vi "relay_block5.vi"(8 "error in":errorcluster, 11 "Modbus master in":refnum<class "Modbus Master.lvclass">) -> (0 "error out":errorcluster, 3 "Modbus master out":refnum<class "Modbus Master.lvclass">)   [LabVIEW 2020]
uses:
  <vilib>/NI/Modbus Library/API/Master/Modbus Master.lvclass
  C:/Program Files/National Instruments/LabVIEW 2020/vi.lib/NI/Modbus Library/API/Modbus API.lvclass
  <vilib>/NI/Modbus Library/API/Modbus API.lvclass/Modbus API.ctl
  <vilib>/NI/Modbus Library/Transmission Data Unit/Transmission Data Unit.lvclass/Transmission Data Unit.ctl
  <vilib>/NI/Modbus Library/Transmission Data Unit/Write Unit ID.vi
  <vilib>/NI/Modbus Library/API/Read Transmission Data Unit.vi
  <vilib>/NI/Modbus Library/API/Write Transmission Data Unit.vi
  status/emergency stop.vi
panel:
  out "current time":timestamp
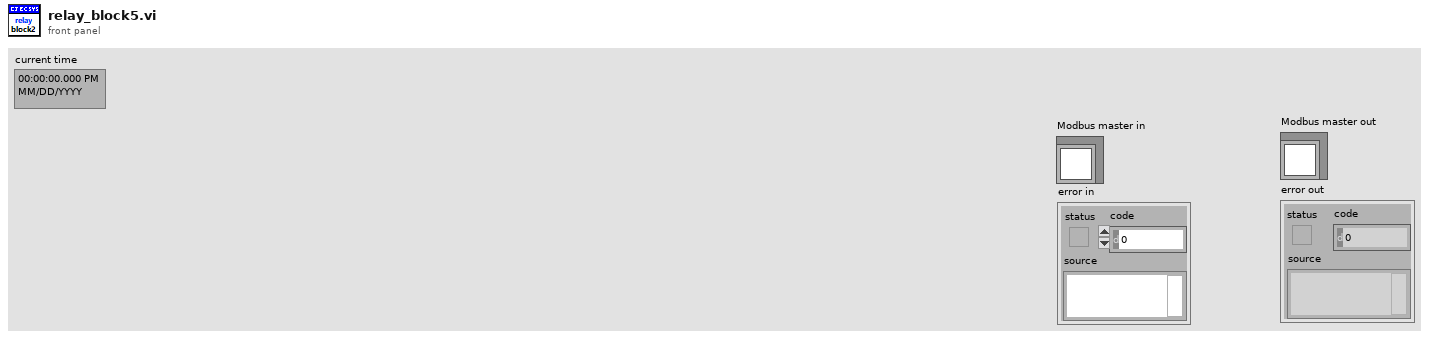
[diagram p1: front panel]
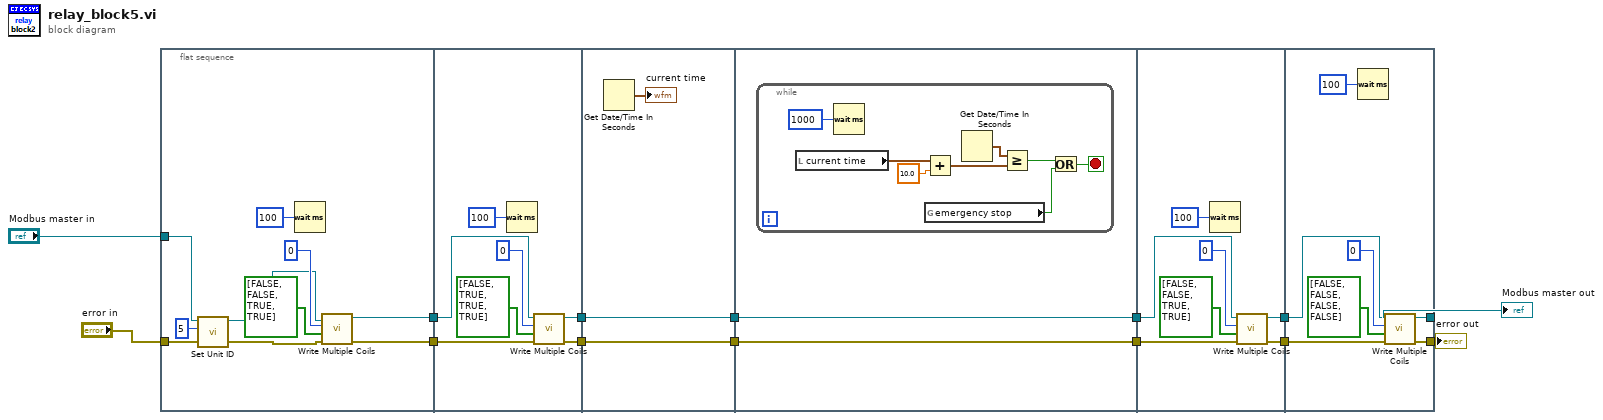
[diagram p0: block diagram]
diagram:
  n1 = flat-sequence {
    tunnel: "error in" -> [w19]
    tunnel: "Modbus master in" -> [w18]
    tunnel: [w21] -> w12
    tunnel: [w20] -> w11
    tunnel: w12 -> [w28]
    tunnel: w11 -> [w27]
    tunnel: [w26] -> w10
    tunnel: [w25] -> w5
    tunnel: w10 -> [w33]
    tunnel: [w33] -> w9
    tunnel: [w32] -> w6
    tunnel: w5 -> [w32]
    tunnel: w9 -> [w36]
    tunnel: [w36] -> w8
    tunnel: [w35] -> w7
    tunnel: w6 -> [w35]
    tunnel: w8 -> [w48]
    tunnel: w7 -> [w47]
    tunnel: [w46] -> w4
    tunnel: [w45] -> w3
    tunnel: w4 -> [w55]
    tunnel: w3 -> [w54]
    tunnel: [w53] -> w2
    tunnel: [w52] -> w1
    frame #0 {
      n2 = call <vilib>:"Set Unit ID.vi"("error in"=w19, "unit ID"=u8 5, "Modbus master in"=w18) -> ("error out"=w16:errorcluster, "Modbus master out"=w17:refnum<class "Modbus Master.lvclass">)  [unwired: 7 in]
      n3 = Wait (ms)(milliseconds to wait=u32 100) -> ()  [unwired: 1 out]
      n4 = call-dynamic "Write Multiple Coils.vi"("error in"=w16, "coils to write"=bool[] [FALSE, FALSE, TRUE, TRUE] ("coils 2"), "starting address"=u16 0, "Modbus master in"=w17) -> ("error out"=w20:errorcluster, "Modbus master out"=w21:refnum<class "Modbus Master.lvclass">)  [unwired: 6 in]
    }
    frame #1 {
      n5 = Wait (ms)(milliseconds to wait=u32 100) -> ()  [unwired: 1 out]
      n6 = call-dynamic "Write Multiple Coils.vi"("error in"=w27, "coils to write"=bool[] [FALSE, TRUE, TRUE, TRUE] ("coils 2"), "starting address"=u16 0, "Modbus master in"=w28) -> ("error out"=w25:errorcluster, "Modbus master out"=w26:refnum<class "Modbus Master.lvclass">)  [unwired: 6 in]
    }
    frame #2 {
      n7 = Get Date/Time In Seconds() -> (seconds since 1Jan1904=→"current time":timestamp)
    }
    frame #3 {
      n8 = while {
        stop <- w37 stop-if-true
        n9 = local read "current time"() -> (w43:timestamp)
        n10 = Wait (ms)(milliseconds to wait=u32 1000 ("millisecond timer value")) -> ()  [unwired: 1 out]
        n11 = Add(x=w43, y=10.0) -> (x+y=w41:timestamp)
        n12 = global read "emergency stop.vi" "emergency stop"() -> (w38:bool)
        n13 = Get Date/Time In Seconds() -> (seconds since 1Jan1904=w40:timestamp)
        n14 = Greater Or Equal?(x=w40, y=w41) -> (x >= y?=w39:bool)
        n15 = Or(x=w39, y=w38) -> (x .or. y?=w37:bool)
      }
    }
    frame #4 {
      n16 = Wait (ms)(milliseconds to wait=u32 100) -> ()  [unwired: 1 out]
      n17 = call-dynamic "Write Multiple Coils.vi"("error in"=w47, "coils to write"=bool[] [FALSE, FALSE, TRUE, TRUE] ("coils 2"), "starting address"=u16 0, "Modbus master in"=w48) -> ("error out"=w45:errorcluster, "Modbus master out"=w46:refnum<class "Modbus Master.lvclass">)  [unwired: 6 in]
    }
    frame #5 {
      n18 = Wait (ms)(milliseconds to wait=u32 100) -> ()  [unwired: 1 out]
      n19 = call-dynamic "Write Multiple Coils.vi"("error in"=w54, "coils to write"=bool[] [FALSE, FALSE, FALSE, FALSE] ("coils 2"), "starting address"=u16 0, "Modbus master in"=w55) -> ("error out"=w52:errorcluster, "Modbus master out"=w53:refnum<class "Modbus Master.lvclass">)  [unwired: 6 in]
    }
  }
  "Modbus master out" <- w2
  "error out" <- w1
